vi "valve_lights.vi"() -> ()   [LabVIEW 2016]
uses:
  <vilib>/DAQmx/read.llb/DAQmx Read (Analog 1D DBL NChan 1Samp).vi
  <vilib>/DAQmx/create/channels.llb/DAQmx Create Channel (AI-Voltage-Basic).vi
  <vilib>/DAQmx/miscellaneous.llb/DAQmx Fill In Error Info.vi
panel:
  out "Open":bool
  out "Closed":bool
  # "Turbo Pump"
  # "Scroll (Roughing) Pump"
  # "Pump"
  # "Back\nPressure\nReadout"
  # "Gate"
  # "Roughing"
  # "Chamber\nPressure\nReadout"
  # "Chamber"
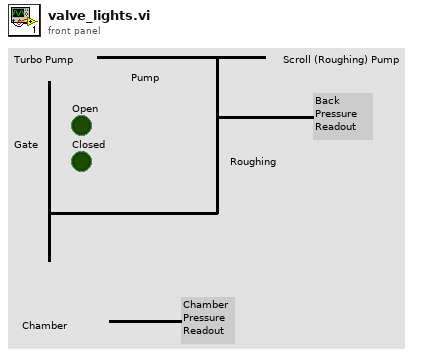
[diagram p1: front panel]
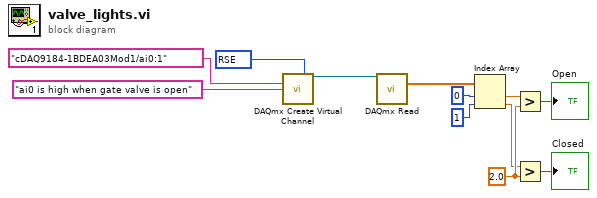
[diagram p0: block diagram]
diagram:
  w8 = 2.0 ("y")
  w12 = 10083 items=["Default"=-1, "RSE"=10083, "NRSE"=10078, "Differential"=10106, "Pseudodifferential"=12529] ("input terminal configuration")
  n1 = call-poly <vilib>:"DAQmx Create Virtual Channel.vi"("input terminal configuration"=w12, "physical channels"=tag "cDAQ9184-1BDEA03Mod1/ai0:1" ("lines"), "name to assign"="ai0 is high when gate valve is open") -> ("task out"=w9:refnum<k21>)  [unwired: 11 in, 1 out]
  n2 = call-poly <vilib>:"DAQmx Read.vi"("task/channels in"=w9) -> ("data"=w5:dbl[])  [unwired: 12 in, 2 out]
  n3 = Index Array(array=w5, index #1=0 ("index"), index #2=1 ("index")) -> (element #1=w4:dbl, element #2=w2:dbl)
  n4 = Greater?(x=w4, y=w8) -> (0:→"Open":bool)
  n5 = Greater?(x=w2, y=w8) -> (0:→"Closed":bool)
